vi "InstrQuery.vi"(8 "error in (no error)":errorcluster, 10 "Command string":string, 11 "InstControl in":refnum<class "InstrControl.lvclass">) -> (0 "error out":errorcluster, 2 "Instrument response":string, 3 "InstControl out":refnum<class "InstrControl.lvclass">)   [LabVIEW 2013, in "InstrControl.lvclass"]
uses:
  InstrControl.lvclass
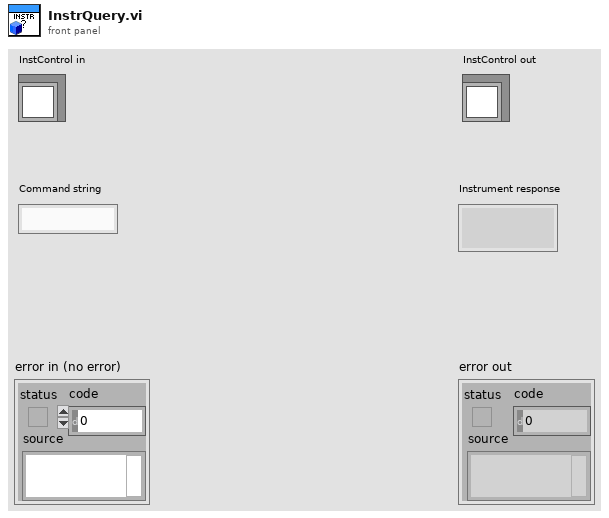
[diagram p1: front panel]
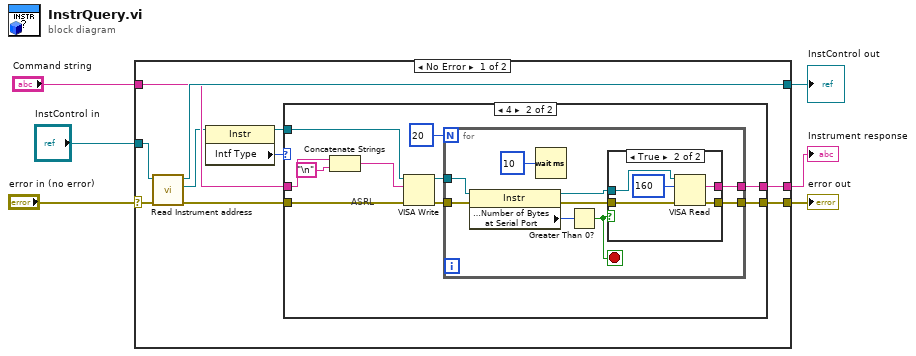
[diagram p0: block diagram]
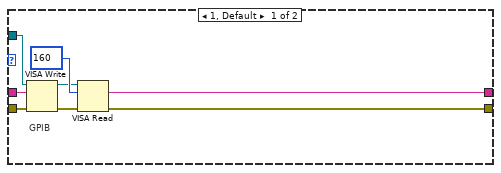
[diagram p2: hidden frame]
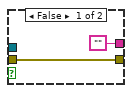
[diagram p3: hidden frame]
diagram:
  n1 = case shown="No Error" "error in (no error)" {
    selector: "error in (no error)" -> [w15 w52]
    tunnel: [w11 w52] -> w5
    tunnel: [w14 w51] -> w3
    tunnel: "InstControl in" -> [w16 w51]
    tunnel: "Command string" -> [w10 _]
    tunnel: [w13 _] -> w1
    frame No Error {
      n2 = call-dynamic "Read Instrument address.vi"("error in (no error)"=w15, "InstControl in"=w16) -> ("error out"=w12:errorcluster, "VISA address"=w9:refnum<visa-resource-name>, "InstControl out"=w14:refnum<class "InstrControl.lvclass">)  [unwired: 7 in]
      n3 = property class="Instr"(reference=w9) -> (reference out=w8:refnum<visa-resource-name>, "Intf Type"=w7:u16)  [unwired: 1 in, 1 out]
      n4 = case shown="4" w7 {
        tunnel: w10 -> [w21 w31]
        tunnel: [w20 w27] -> w13
        tunnel: w12 -> [w19 w34]
        tunnel: w8 -> [w18 w33]
        tunnel: [w17 w26] -> w11
        frame 1, Default {
          # "GPIB"
          n5 = VISA Write(VISA resource name=w18, write buffer=w21, error in (no error)=w19) -> (VISA resource name out=w23:refnum<visa-resource-name>, error out=w22:errorcluster)  [unwired: 1 out]
          n6 = VISA Read(VISA resource name=w23, byte count=160, error in (no error)=w22) -> (read buffer=w20:string, error out=w17:errorcluster)  [unwired: 2 out]
        }
        frame 4 {
          # "ASRL"
          n7 = Concatenate Strings(w31, "\n") -> (w30:string)
          n8 = VISA Write(VISA resource name=w33, write buffer=w30, error in (no error)=w34) -> (VISA resource name out=w29:refnum<visa-resource-name>, error out=w28:errorcluster)  [unwired: 1 out]
          n9 = for {
            N: 20 -> [_]
            tunnel: [w41] -> w27
            tunnel: w29 -> [w37]
            tunnel: [w40] -> w26
            tunnel: w28 -> [w38]
            stop <- w35 stop-if-true
            n10 = property class="Instr"(reference=w37, error in=w38) -> (reference out=w43:refnum<visa-resource-name>, error out=w42:errorcluster, "Serial Settings:Number of Bytes at Serial Port"=w36:u32)
            n11 = Wait (ms)(milliseconds to wait=10) -> ()  [unwired: 1 out]
            n12 = Greater Than 0?(x=w36) -> (x > 0?=w35:bool)
            n13 = case shown="True" w35 {
              tunnel: w43 -> [_ w50]
              tunnel: w42 -> [w44 w49]
              tunnel: ["" w48] -> w41
              tunnel: [w44 w47] -> w40
              frame False {
              }
              frame True {
                n14 = VISA Read(VISA resource name=w50, byte count=160, error in (no error)=w49) -> (read buffer=w48:string, error out=w47:errorcluster)  [unwired: 2 out]
              }
            }
          }
        }
      }
    }
    frame Error {
    }
  }
  "error out" <- w5
  "InstControl out" <- w3
  "Instrument response" <- w1
